vi "Create Conpane Image File.vi"(8 "error in":errorcluster, 9 "Name":string, 10 "Conpane Image":T1, 11 "Image Folder Path":path) -> (0 "error out":errorcluster, 3 "File Name":string)   [LabVIEW 2021, in "TAF Proj Document Type.lvlib"]
uses:
  <vilib>/Wovalab/AntiDoc/Document Type/Add-ons/LabVIEW TAF Project/TAF Proj Document Type.lvlib
  <vilib>/picture/picture.llb/imagedata.ctl
  <vilib>/Wovalab/AntiDoc/Utilities/Utilities.lvlib
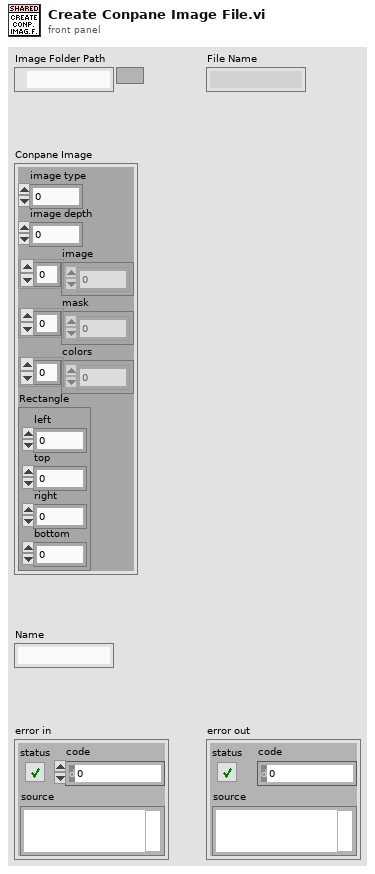
[diagram p1: front panel]
types:
  T1 = typedef "imagedata.ctl" = cluster{"image type":i32, "image depth":i32, "image":u8[], "mask":u8[], "colors":u32[], "Rectangle":cluster{"left":i16, "top":i16, "right":i16, "bottom":i16}}
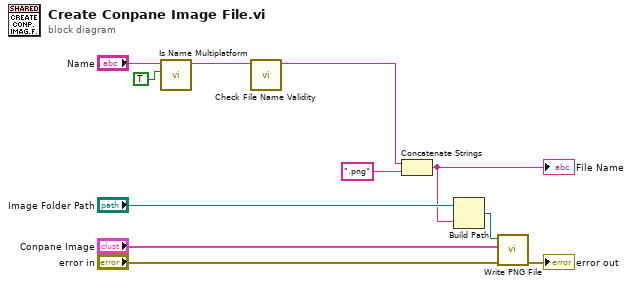
[diagram p0: block diagram]
diagram:
  n1 = call <vilib>:"Is Name Multiplatform.vi"("filename must be valid on all platforms (F)"=TRUE, "filename"="Name") -> ("suggested filename"=w2:string)  [unwired: 5 in, 4 out]
  n2 = call <vilib>:"Check File Name Validity.vi"("Path in"=w2) -> ("Path out"=w1:string)  [unwired: 10 in]
  n3 = Concatenate Strings(w1, ".png" ("string")) -> (w8:string)
  "File Name" <- w8
  n4 = Build Path(base path="Image Folder Path", name or relative path=w8) -> (appended path=w6:path)
  n5 = call <vilib>:"Write PNG File.vi"("error in (no error)"="error in", "image data"="Conpane Image", "path to PNG file"=w6) -> ("error out"=→"error out":errorcluster)  [unwired: 7 in, 1 out]
